vi "WiFi SoftAP Example.vi"   [LabVIEW 2014]
uses:
  QwaveSys_ESP8266/QwaveSys_ESP8266.lvlib
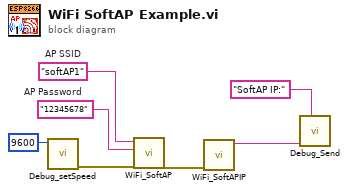
[diagram p0: block diagram]
diagram:
  w5 = "12345678"  # AP Password
  w6 = "softAP1"  # AP SSID
  n1 = call "Debug_setSpeed.vi"("Speed"=u32 9600) -> ("error out"=w2:errorcluster)  [unwired: 10 in]
  n2 = call "WiFi_SoftAP.vi"("error in (no error)"=w2, "AP Password"=w5, "AP SSID"=w6) -> ("error out"=w7:errorcluster)  [unwired: 8 in]
  n3 = call "WiFi_SoftAPIP.vi"("error in (no error)"=w7) -> ("IP"=w4:string)  [unwired: 9 in, 1 out]
  n4 = call "Debug_Send.vi"("Name"="SoftAP IP:", "DATA"=w4) -> ()  [unwired: 10 in]
